vi "Smooth.vi"(10 "x":dbl) -> (2 "y":dbl)   [LabVIEW 2015]
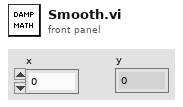
[diagram p1: front panel]
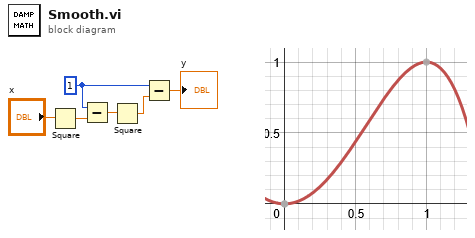
[diagram p0: block diagram]
diagram:
  w3 = 1
  n1 = Square(x="x") -> (x^2=w5:dbl)
  n2 = Subtract(x=w3, y=w5) -> (x-y=w4:dbl)
  n3 = Square(x=w4) -> (x^2=w2:dbl)
  n4 = Subtract(x=w3, y=w2) -> (x-y=→"y":dbl)
